vi "waitUntilStarted.vi"(8 "error in (no error)":errorcluster, 11 "CameraManager in":refnum<class "CameraManager.lvclass">) -> (0 "error out":errorcluster, 3 "CameraManager out":refnum<class "CameraManager.lvclass">)   [LabVIEW 2011, in "iManagement.lvlib" / "CameraManager.lvclass"]
uses:
  CameraManager.lvclass
  CameraManager.lvclass/CameraManager.ctl
  Hal/Channels/Camera/CameraController.lvclass
  Hal/Channels/Camera/CameraEventsManager/CameraEventsManger.lvclass
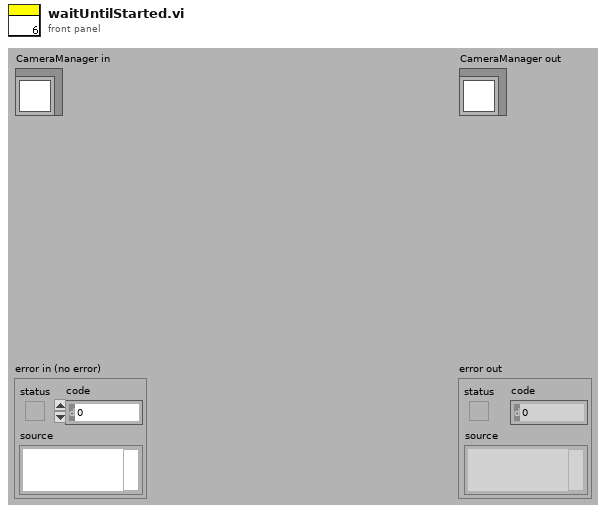
[diagram p1: front panel]
types:
  T1 = cluster{"settingsFrontEndEvents":cluster{"loadSettingsFromPath":refnum<user-event>, "lookUpElementEvent":refnum<user-event>, "saveSettings":refnum<user-event>, "loadSettings":refnum<user-event>, "close":refnum<user-event>, "replaceElement":refnum<user-event>, "findParentNodes":refnum<user-event>, "createNode":refnum<user-event>}, "settingBackEndEvents":cluster{"defaultSettingsPathRequest":refnum<user-event>, "searchResultEvent":refnum<user-event>, "settingsSaved":refnum<user-event>, "settingsLoaded":refnum<user-event>, "foundParentNode":refnum<user-event>}}
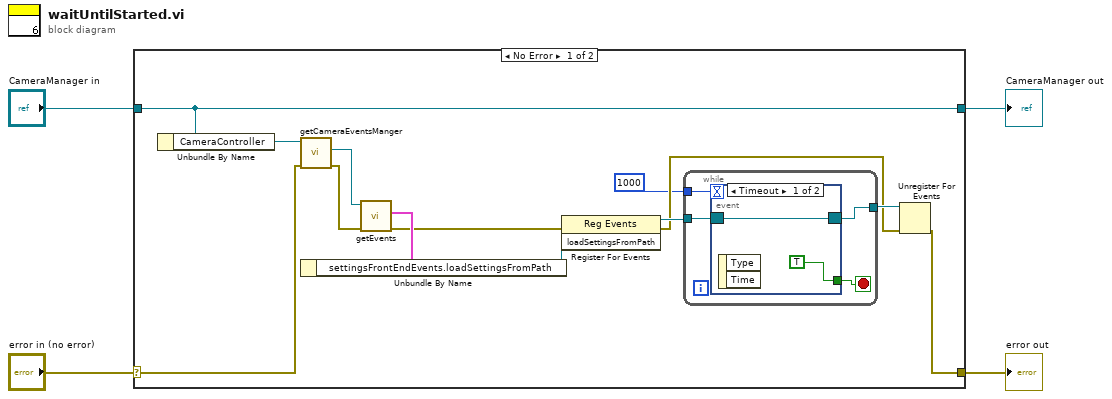
[diagram p0: block diagram]
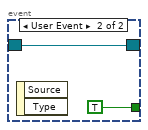
[diagram p2: hidden frame]
diagram:
  n1 = case shown="No Error" "error in (no error)" {
    selector: "error in (no error)" -> [w13 w27]
    tunnel: [w7 w27] -> w3
    tunnel: [w17 w26] -> w1
    tunnel: "CameraManager in" -> [w17 w26]
    frame No Error {
      n2 = Unbundle By Name(w17) -> ("CameraController"=w16:refnum<class "CameraController.lvclass">)
      n3 = call-dynamic "getCameraEventsManger.vi"("error in (no error)"=w13, "CameraController.lvclass in"=w16) -> ("error out"=w14:errorcluster, "Hardware:Channels.lvlib:CameraEventsManger.lvclass"=w15:refnum<class "CameraEventsManger.lvclass">)  [unwired: 7 in, 1 out]
      n4 = call-dynamic "getEvents.vi"("error in (no error)"=w14, "CameraEventsManger in"=w15) -> ("error out"=w6:errorcluster, "settingsEvents"=w12:T1)  [unwired: 5 in, 3 out]
      n5 = Unbundle By Name(w12) -> ("settingsFrontEndEvents.loadSettingsFromPath"=w11:refnum<user-event>)
      n6 = register-events(error in=w6, w11) -> (reference out=w10:refnum<event-registration>, error out=w8:errorcluster)  [unwired: 1 in]
      n7 = while {
        tunnel: w10 -> [w21]
        tunnel: [w19] -> w9
        tunnel: 1000 -> [w18]
        stop <- w20 stop-if-true
        n8 = event shown="[0] Timeout" {
          selector: w21 -> [w23 w24]
          dyn-events: [w23 w24] -> w19
          timeout: w18 -> [_ _]
          tunnel: [TRUE TRUE] -> w20
          event Timeout {
            n9 = event-data() -> ()  [unwired: 1 in, 2 out]
          }
          event User Event {
            n10 = event-data() -> ()  [unwired: 1 in, 2 out]
          }
        }
      }
      n11 = Unregister For Events(event registration refnum=w9, error in=w8) -> (error out=w7:errorcluster)
    }
    frame Error {
    }
  }
  "error out" <- w3
  "CameraManager out" <- w1
